vi "CS++CoreContent.vi"   [LabVIEW 2014]
doc: "Place actor and class constants that should be included included in an application on the blockdiagramm."
uses:
  Actors/CS++StartActor/CS++StartActor.lvclass
  Actors/CS++BaseActor/CS++BaseActor.lvclass
  Actors/CS++PVMonitor/CS++PVMonitor.lvclass
  Actors/CS++SVMonitor/CS++SVMonitor.lvclass
  Actors/CS++ControllerActor/CS++ControllerActor.lvclass
  Actors/CS++DeviceActor/CS++DeviceActor.lvclass
  Classes/CS++BaseClasses/Base/CS++Base.lvclass
  Classes/CS++BaseClasses/Factory/CS++Factory.lvclass
  Classes/CS++BaseClasses/Reference/CS++Reference.lvclass
  Classes/CS++ProcessVariables/ProcessVariable/PV.lvclass
  Classes/CS++ProcessVariables/PVConnection/PVConnection.lvclass
  Classes/CS++ProcessVariables/SVConnection/SVConnection.lvclass
  Classes/CS++BaseClasses/MessageLogger/CS++MessageLogger.lvclass
panel:
  # "Place actor and class constants on the blockdiagramm."
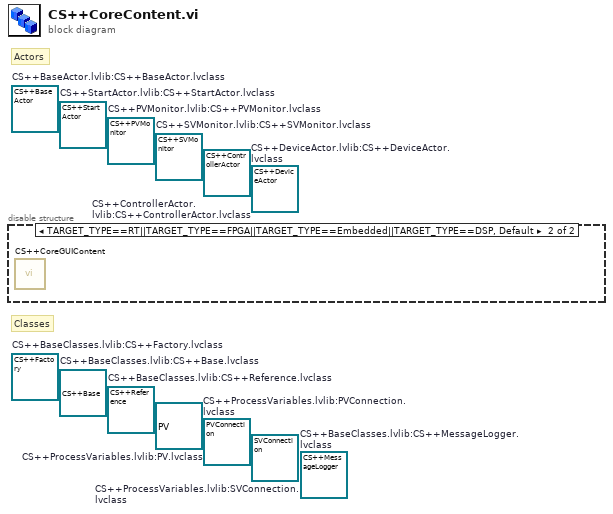
[diagram p0: block diagram]
diagram:
  (unwired) refnum<class "CS++MessageLogger.lvclass"> refnum  # CS++BaseClasses.lvlib:CS++MessageLogger.lvclass
  (unwired) refnum<class "SVConnection.lvclass"> refnum  # CS++ProcessVariables.lvlib:SVConnection.lvclass
  (unwired) refnum<class "PVConnection.lvclass"> refnum  # CS++ProcessVariables.lvlib:PVConnection.lvclass
  (unwired) refnum<class "PV.lvclass"> refnum  # CS++ProcessVariables.lvlib:PV.lvclass
  (unwired) refnum<class "CS++Reference.lvclass"> refnum  # CS++BaseClasses.lvlib:CS++Reference.lvclass
  (unwired) refnum<class "CS++Factory.lvclass"> refnum  # CS++BaseClasses.lvlib:CS++Factory.lvclass
  (unwired) refnum<class "CS++Base.lvclass"> refnum  # CS++BaseClasses.lvlib:CS++Base.lvclass
  (unwired) refnum<class "CS++DeviceActor.lvclass"> refnum  # CS++DeviceActor.lvlib:CS++DeviceActor.lvclass
  (unwired) refnum<class "CS++ControllerActor.lvclass"> refnum  # CS++ControllerActor.lvlib:CS++ControllerActor.lvclass
  (unwired) refnum<class "CS++SVMonitor.lvclass"> refnum  # CS++SVMonitor.lvlib:CS++SVMonitor.lvclass
  (unwired) refnum<class "CS++PVMonitor.lvclass"> refnum  # CS++PVMonitor.lvlib:CS++PVMonitor.lvclass
  (unwired) refnum<class "CS++BaseActor.lvclass"> refnum  # CS++BaseActor.lvlib:CS++BaseActor.lvclass
  (unwired) refnum<class "CS++StartActor.lvclass"> refnum  # CS++StartActor.lvlib:CS++StartActor.lvclass
  # "Classes"
  # "Actors"
  n1 = disable-structure shown="TARGET_TYPE==RT||TARGET_TYPE==FPGA||TARGET_TYPE==Embedded||TARGET_TYPE==DSP, Default" {
    frame condition #0 (active) {
    }
    frame condition #1 {
      n2 = call "CS++CoreGUIContent.vi"() -> ()  [unwired: 12 in]
    }
  }
